vi "Update Data Record On Disk.vi"(0 "Graph Entry":T1) -> ()   [LabVIEW 2013]
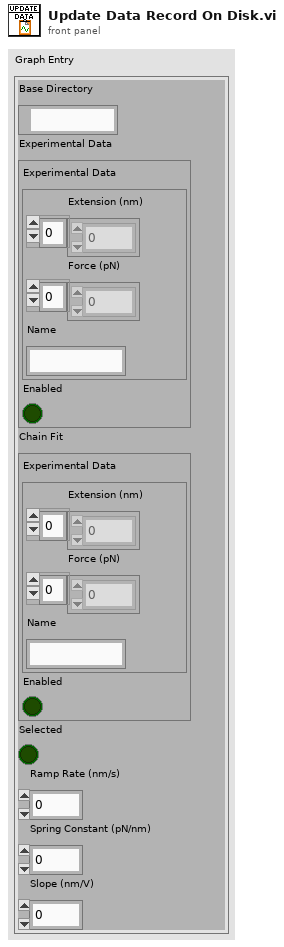
[diagram p1: front panel]
types:
  T1 = cluster{"Base Directory":path, "Experimental Data":cluster{"Experimental Data":cluster{"Extension (nm)":dbl[], "Force (pN)":dbl[], "Name":string}, "Enabled":bool}, "Chain Fit":cluster{"Experimental Data":cluster{"Extension (nm)":dbl[], "Force (pN)":dbl[], "Name":string}, "Enabled":bool}, "Selected":bool, "Ramp Rate (nm/s)":dbl, "Spring Constant (pN/nm)":dbl, "Slope (nm/V)":dbl}
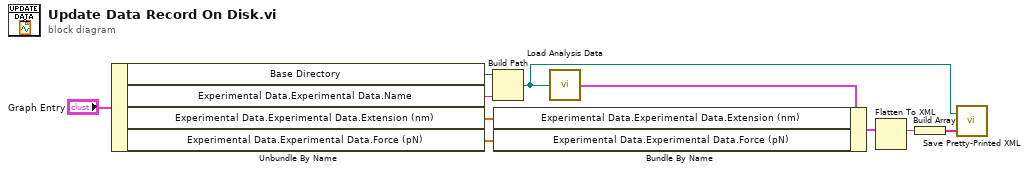
[diagram p0: block diagram]
diagram:
  n1 = Unbundle By Name("Graph Entry") -> ("Base Directory"=w8:path, "Experimental Data.Experimental Data.Name"=w9:string, "Experimental Data.Experimental Data.Extension (nm)"=w6:dbl[], "Experimental Data.Experimental Data.Force (pN)"=w5:dbl[])
  n2 = Build Path(base path=w8, name or relative path=w9) -> (appended path=w1:path)
  n3 = call "Load Analysis Data.vi"("Load Path"=w1) -> ("Loaded Entry"=w7:T1)
  n4 = Bundle By Name(cluster=w7, "Experimental Data.Experimental Data.Extension (nm)"=w6, "Experimental Data.Experimental Data.Force (pN)"=w5) -> (w4:T1)
  n5 = Flatten To XML(anything=w4) -> (xml string=w3:string)
  n6 = Build Array(w3) -> (w2:string[])
  n7 = call "Save Pretty-Printed XML.vi"("XML Input"=w2, "XML File Path"=w1) -> ()
